vi "Get Forecast Current Data.vi"(8 "error in (no error)":errorcluster, 11 "API Output":string) -> (0 "error out":errorcluster, 2 "Current Data":T1 {"currently"."time" format="%#_10g"}, 3 "API Output (copy)":string)   [LabVIEW 2017, in "Dark Sky Weather Data for LabVIEW.lvlib"]
doc: "Parses the Dark Sky API's output for current weather conditions."
uses:
  Dark Sky Weather Data for LabVIEW.lvlib
  Controls/Forecast Current Data.ctl
  <vilib>/addons/_JKI.lib/Serialization/JSON/JKI JSON Serialization.lvlib
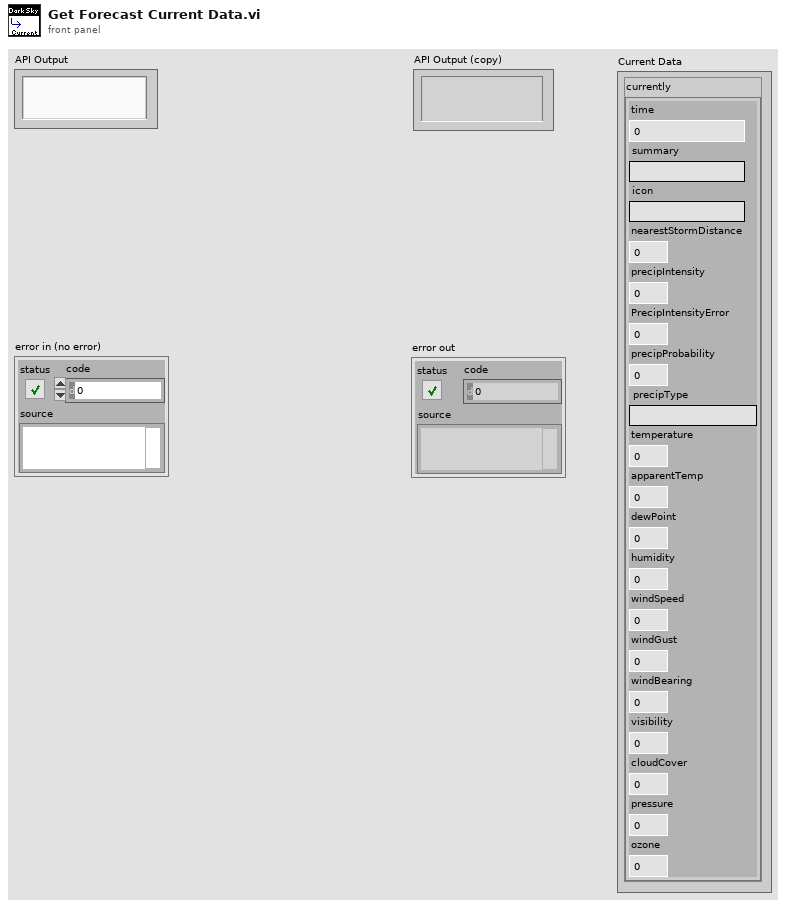
[diagram p1: front panel]
types:
  T1 = typedef "Dark Sky Weather Data for LabVIEW.lvlib/Forecast Current Data.ctl" = cluster{"currently":cluster{"time":dbl, "summary":string, "icon":string, "nearestStormDistance":dbl, "precipIntensity":dbl, "PrecipIntensityError":dbl, "precipProbability":dbl, "precipType":string, "temperature":dbl, "apparentTemp":dbl, "dewPoint":dbl, "humidity":dbl, "windSpeed":dbl, "windGust":dbl, "windBearing":dbl, "visibility":dbl, "cloudCover":dbl, "pressure":dbl, "ozone":dbl}}
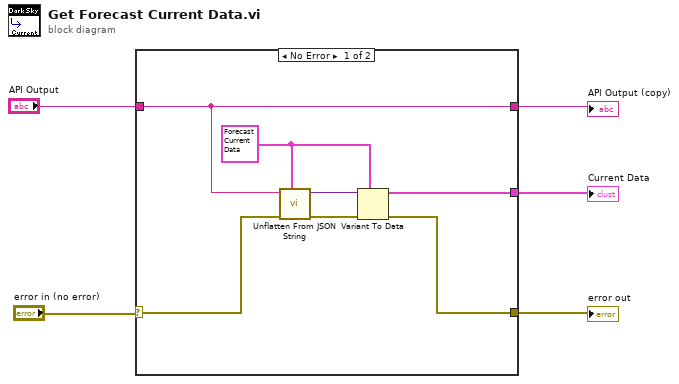
[diagram p0: block diagram]
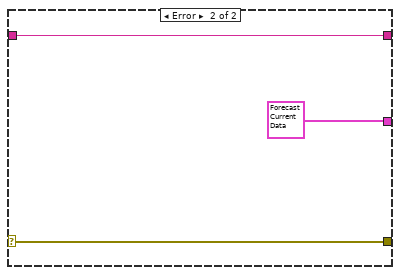
[diagram p2: hidden frame]
diagram:
  n1 = case shown="No Error" "error in (no error)" {
    selector: "error in (no error)" -> [w12 w15]
    tunnel: [w9 w15] -> w4
    tunnel: "API Output" -> [w7 w14]
    tunnel: [w8 T1 {"currently"={"time"=0.0, "summary"="", "icon"="", "nearestStormDistance"=0.0, "precipIntensity"=0.0, "PrecipIntensityError"=0.0, "precipProbability"=0.0, "precipType"="", "temperature"=0.0, "apparentTemp"=0.0, "dewPoint"=0.0, "humidity"=0.0, "windSpeed"=0.0, "windGust"=0.0, "windBearing"=0.0, "visibility"=0.0, "cloudCover"=0.0, "pressure"=0.0, "ozone"=0.0}} ("currently")] -> w1
    tunnel: [w7 w14] -> w2
    frame No Error {
      w6 = T1 {"currently"={"time"=0.0, "summary"="", "icon"="", "nearestStormDistance"=0.0, "precipIntensity"=0.0, "PrecipIntensityError"=0.0, "precipProbability"=0.0, "precipType"="", "temperature"=0.0, "apparentTemp"=0.0, "dewPoint"=0.0, "humidity"=0.0, "windSpeed"=0.0, "windGust"=0.0, "windBearing"=0.0, "visibility"=0.0, "cloudCover"=0.0, "pressure"=0.0, "ozone"=0.0}} ("currently")
      n2 = call <vilib>:"Unflatten From JSON String.vi"("Type and Defaults"=w6, "error in (no error)"=w12, "JSON String"=w7) -> ("error out"=w10:errorcluster, "Variant"=w11:variant)  [unwired: 7 in]
      n3 = Variant To Data(error in=w10, type=w6, Variant=w11) -> (data=w8:T1, error out=w9:errorcluster)
    }
    frame Error {
    }
  }
  "error out" <- w4
  "API Output (copy)" <- w2
  "Current Data" <- w1
